vi "Pic with Bird (SubVI).vi"(9 "Bird Position":dbl format="%.2f", 10 "X position":i32, 11 "Picture in":i32[][](array[numeric])=array200x100[20000 elements]) -> (3 "Picture":i32[][](array[numeric]))   [LabVIEW 2013]
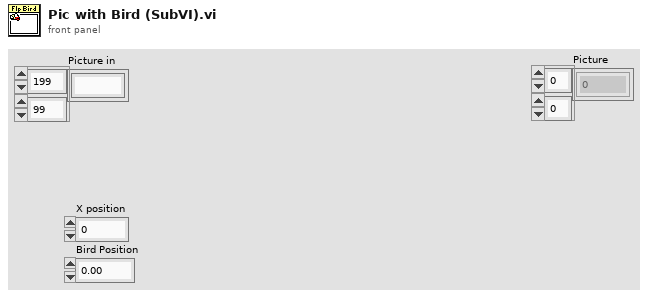
[diagram p1: front panel]
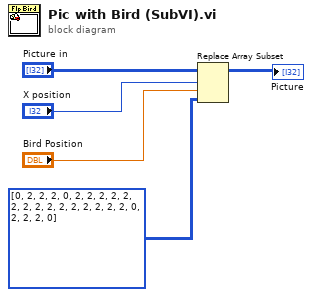
[diagram p0: block diagram]
diagram:
  n1 = Replace Array Subset(array="Picture in", new element=i32[][] [[0, 2, 2, 2, 0], [2, 2, 2, 2, 2], [2, 2, 2, 2, 2], [2, 2, 2, 2, 2], [0, 2, 2, 2, 0]] ("Picture in"), index (row)="X position", index (col)="Bird Position") -> (→"Picture":i32[][])
